vi "EmuladorTest_subVI.vi"(4 "START":bool, 6 "cancel test":bool, 7 "Datos_QR":string, 9 "Operator's name":string, 10 "Config File":path, 11 "Path Out Report":path) -> (2 "Boolean":bool=TRUE)   [LabVIEW 2019]
panel:
  out "cancel test 2":bool
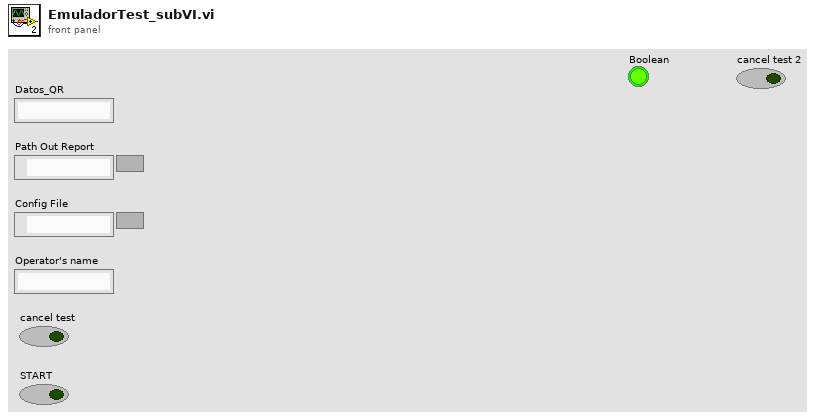
[diagram p1: front panel]
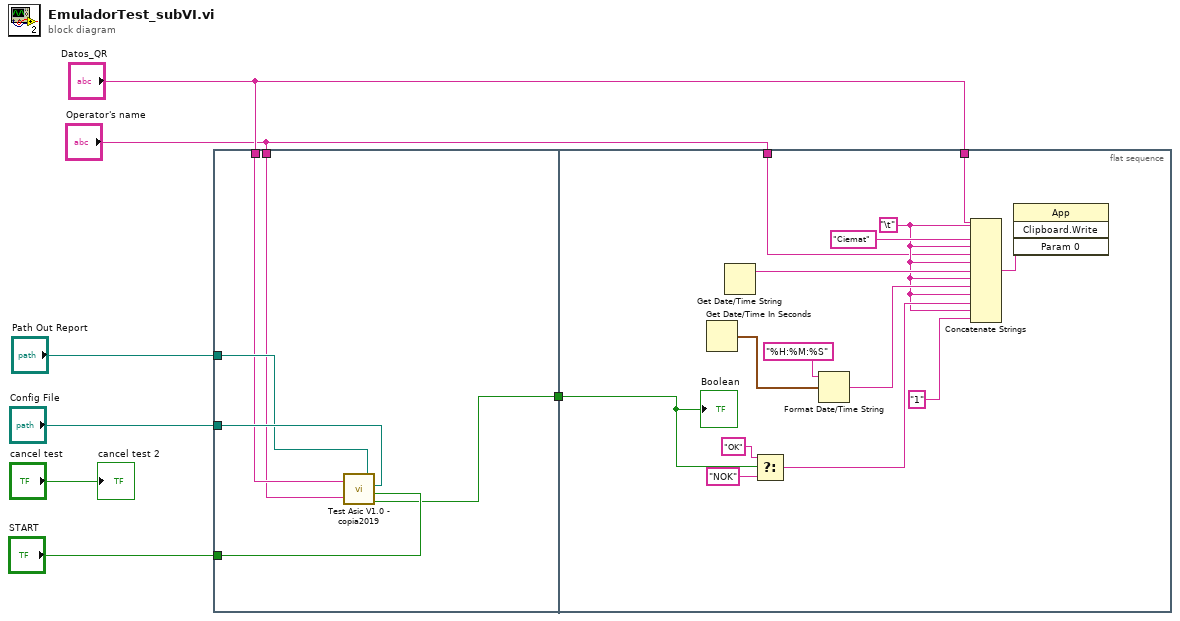
[diagram p0: block diagram]
diagram:
  n1 = flat-sequence {
    tunnel: [w8] -> w6
    tunnel: "Config File" -> [w13]
    tunnel: "START" -> [w12]
    tunnel: "Path Out Report" -> [w11]
    tunnel: "Datos_QR" -> [w10]
    tunnel: "Operator's name" -> [w9]
    tunnel: w6 -> [w25]
    tunnel: "Datos_QR" -> [w15]
    tunnel: "Operator's name" -> [w14]
    frame #0 {
      n2 = call "Test Asic V1.0 - copia2019.vi"("ASIC'S Number"=w10, "Operator's Name"=w9, "Path Out Report"=w11, "Config File"=w13, "START"=w12) -> ("OK, Fault 2"=w8:bool)
    }
    frame #1 {
      w16 = "\t"
      n3 = Get Date/Time In Seconds() -> (seconds since 1Jan1904=w23:timestamp)
      n4 = Get Date/Time String() -> (date string=w20:string)  [unwired: 3 in, 1 out]
      n5 = Select(t="OK", s=w25, f="NOK") -> (s? t:f=w18:string)
      n6 = Format Date/Time String(time format string (%c)="%H:%M:%S", seconds (now)=w23) -> (date/time string=w19:string)  [unwired: 1 in]
      n7 = Concatenate Strings(w15, w16, "Ciemat", w16, w14, w16, w20, w16, w19, w16, w18, w16, "1") -> (w24:string)
      n8 = invoke class="App" method="Clipboard.Write"("Param 0"=w24) -> ()  [unwired: 3 in, 4 out]
      "Boolean" <- w25
    }
  }
  "cancel test 2" <- "cancel test"
